vi "20170509-lecture4-2 buttons.vi"() -> ()   [LabVIEW 2014]
panel:
  out "array":bool[](array[boolean])
  in  "stop":bool
  in  "Master Cluster":T1
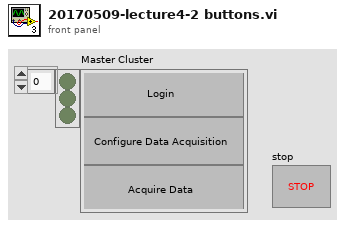
[diagram p1: front panel]
types:
  T1 = cluster{"Login":bool, "Configure Data Acquisition":bool, "Acquire Data":bool}
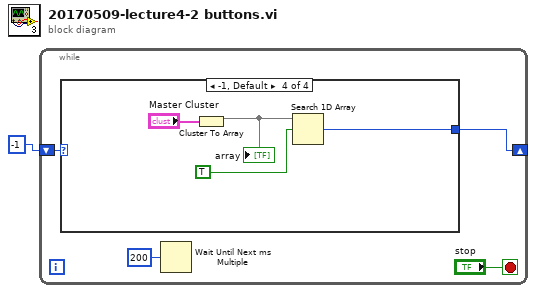
[diagram p0: block diagram]
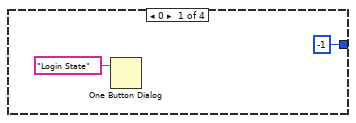
[diagram p2: hidden frame]
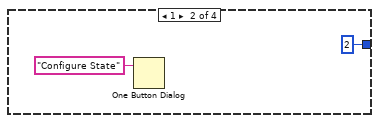
[diagram p3: hidden frame]
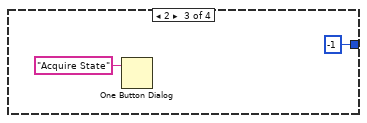
[diagram p4: hidden frame]
diagram:
  n1 = while {
    shift-right: [w3] -> _
    shift-left: -1 -> [w4]
    stop <- "stop" stop-if-true
    n2 = case shown="-1, Default" w4 {
      tunnel: [-1 ("index of element") 2 ("index of element") -1 ("index of element") w12] -> w3
      frame 0 {
        n3 = One Button Dialog(message="Login State") -> ()  [unwired: 1 in, 1 out]
      }
      frame 1 {
        n4 = One Button Dialog(message="Configure State") -> ()  [unwired: 1 in, 1 out]
      }
      frame 2 {
        n5 = One Button Dialog(message="Acquire State") -> ()  [unwired: 1 in, 1 out]
      }
      frame -1, Default {
        n6 = Cluster To Array(cluster="Master Cluster") -> (array=w14:bool[])
        "array" <- w14
        n7 = Search 1D Array(1D array=w14, element=TRUE) -> (index of element=w12:i32)  [unwired: 1 in]
      }
    }
    n8 = Wait Until Next ms Multiple(millisecond multiple=u32 200) -> ()  [unwired: 1 out]
  }
